vi "AI FSM.vi"(8 "Error In":errorcluster, 11 "Robot Mode":T1(ring)) -> (0 "Error Out":errorcluster, 1 "Heading_Cmd":dbl, 2 "VTan_Cmd":dbl, 3 "VAng_Cmd":dbl)   [LabVIEW 2012]
uses:
  Utilities/Robot Parameters/Robot Parameters.vi
panel:
  out "Bearing":dbl
  out "Target Distance":dbl
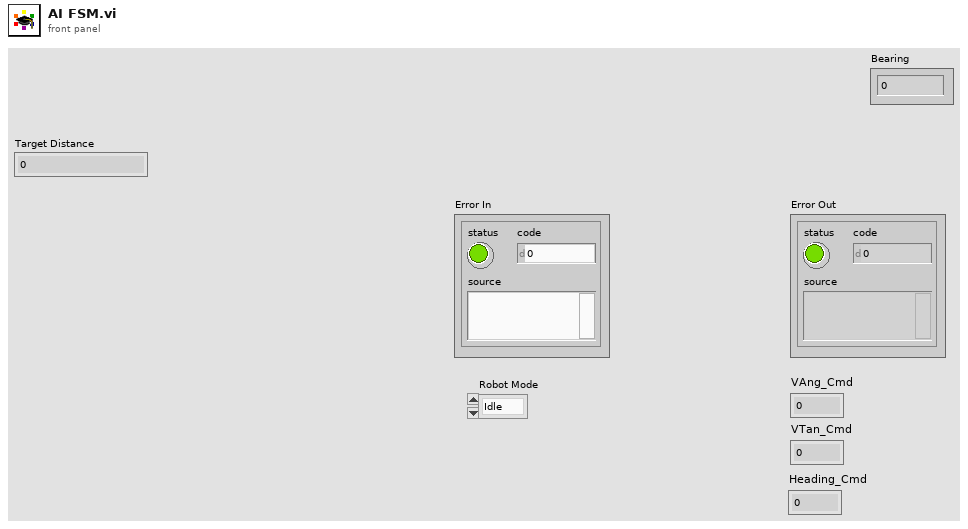
[diagram p1: front panel]
types:
  T1 = enum16{"Idle", "Wiimote", "Joypad", "IGVC", "Avoide Objects", "Avoide Lines", "Path Planning", "Heading", "Waypoint"}
  T2 = enum16{"Starting Line", "Line Following", "Waypoint Navigation", "Fence Hopping", "Finish Line", "Emergency"}
  T3 = cluster{"Latitude":dbl, "Longitude":dbl, "Altitude":dbl, "Velocity, Correction & SET":cluster{"Velocity North":dbl, "Velocity East":dbl, "Velocity Up":dbl, "Ellipsoidal Height":dbl, "GDOP":sgl, "PDOP":sgl, "HDOP":sgl, "VDOP":sgl, "TDOP":sgl, "Horizontal Figure of Merit":u8, "Time Figure of Merit":u8, "Max dGPS Age":sgl, "Extended Navigation Mode":u8, "Antenna Height Adjustment ":dbl, "SET North":i32, "SET East":i32, "SET Up":i32}, "Time":cluster{"GPS Week":u16, "GPS Time of Week":sgl}, "Satellites Used":i32[]}
  T4 = cluster{"Position":cluster{"Roll":dbl, "Pitch":dbl, "Yaw":dbl}, "Orientation Matrix":dbl[][], "Magnetic Field":cluster{"Z-Axis Magnetic Field":dbl, "Y-Axis Magnetic Field":dbl, "X-Axis Magnetic Field":dbl}, "Acceleration":cluster{"Z-Axis Acceleration":dbl, "Y-Axis Acceleration":dbl, "X-Axis Acceleration":dbl}, "Angular Rate":cluster{"X-Axis Angular Rate":dbl, "Y-Axis Angular Rate":dbl, "Z-Axis Angular Rate":dbl}, "Quaternion":dbl[]}
  T5 = cluster{"Latitude":dbl, "Longitude":dbl, "Altitude":dbl, "Velocity, Correction & SET":cluster{"Velocity North":dbl, "Velocity East":dbl, "Velocity Up":dbl, "Ellipsoidal Height":dbl, "GDOP":sgl, "PDOP":sgl, "HDOP":sgl, "VDOP":sgl, "TDOP":sgl, "Horizontal Figure of Merit":u8, "Time Figure of Merit":u8, "Max dGPS Age":sgl, "Extended Navigation Mode":u8, "Antenna Height Adjustment ":dbl, "SET North":i32, "SET East":i32, "SET Up":i32}, "Time":cluster{"GPS Week":u16, "GPS Time of Week":sgl}, "Satellites Used":i32[]}[]
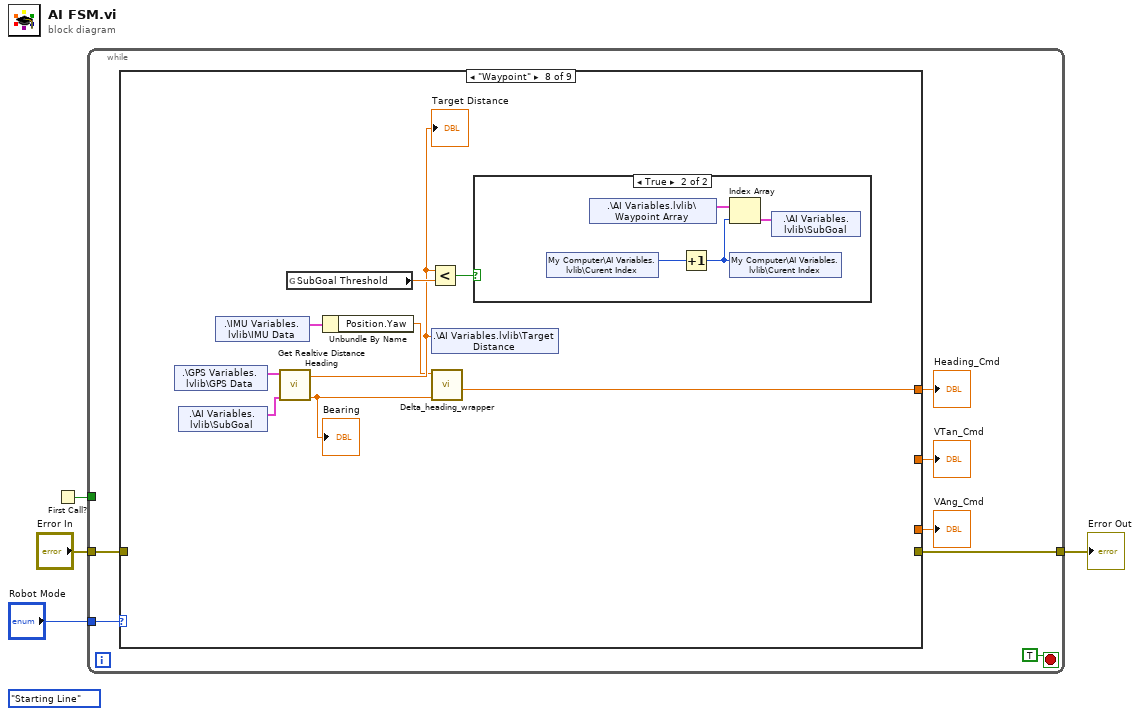
[diagram p0: block diagram]
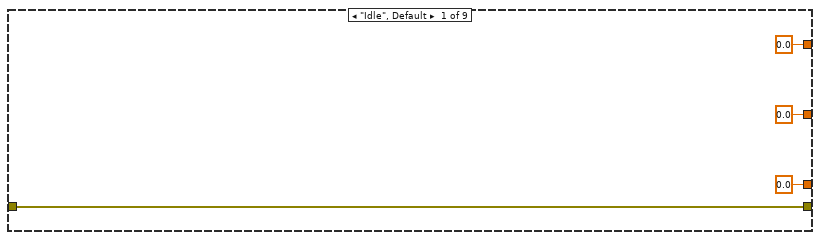
[diagram p2: hidden frame]
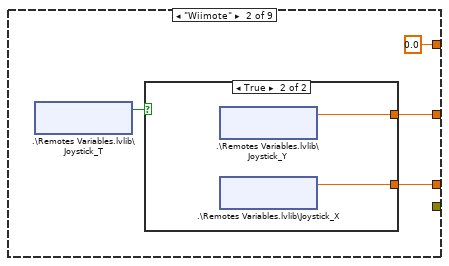
[diagram p3: hidden frame]
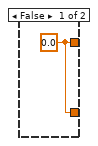
[diagram p4: hidden frame]
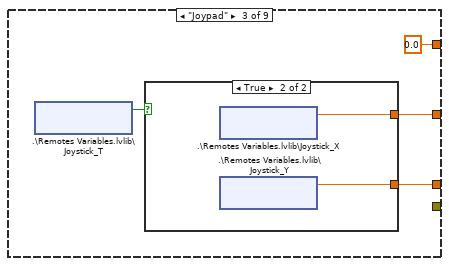
[diagram p5: hidden frame]
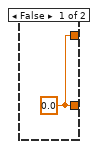
[diagram p6: hidden frame]
diagram:
  (unwired) T2."Starting Line" ("Enum")
  n1 = First Call?() -> (First Call?: T/F=w4:bool)
  n2 = while {
    tunnel: w4 -> [_]
    tunnel: "Error In" -> [w9]
    tunnel: [w8] -> w2
    tunnel: "Robot Mode" -> [w10]
    stop <- TRUE stop-if-true
    n3 = case shown="\"Waypoint\"" w10 {
      tunnel: [0.0 0.0 ("Numeric") 0.0 ("Numeric") _ _ _ _ w32 _] -> w5
      tunnel: [0.0 ("Double") w18 w23 _ _ _ _ _ _] -> w7
      tunnel: [0.0 w17 w25 _ _ _ _ _ _] -> w6
      tunnel: w9 -> [w13 _ _ _ _ _ _ _ _]
      tunnel: [w13 _ _ _ _ _ _ _ _] -> w8
      frame "Idle", Default {
      }
      frame "Wiimote" {
        n4 = shared-variable ".\\Remotes Variables.lvlib\\Joystick_T"() -> (w19:bool)  [unwired: 1 in, 2 out]
        n5 = case shown="True" w19 {
          tunnel: [w20 w22] -> w18
          tunnel: [w20 w21] -> w17
          frame False {
            w20 = 0.0
          }
          frame True {
            n6 = shared-variable ".\\Remotes Variables.lvlib\\Joystick_Y"() -> (w22:dbl)  [unwired: 1 in, 2 out]
            n7 = shared-variable ".\\Remotes Variables.lvlib\\Joystick_X"() -> (w21:dbl)  [unwired: 1 in, 2 out]
          }
        }
      }
      frame "Joypad" {
        n8 = shared-variable ".\\Remotes Variables.lvlib\\Joystick_T"() -> (w26:bool)  [unwired: 1 in, 2 out]
        n9 = case shown="True" w26 {
          tunnel: [w27 w29] -> w25
          tunnel: [w27 w28] -> w23
          frame False {
            w27 = 0.0
          }
          frame True {
            n10 = shared-variable ".\\Remotes Variables.lvlib\\Joystick_X"() -> (w28:dbl)  [unwired: 1 in, 2 out]
            n11 = shared-variable ".\\Remotes Variables.lvlib\\Joystick_Y"() -> (w29:dbl)  [unwired: 1 in, 2 out]
          }
        }
      }
      frame "IGVC" {
      }
      frame "Avoide Objects" {
      }
      frame "Avoide Lines" {
      }
      frame "Heading" {
      }
      frame "Waypoint" {
        n12 = shared-variable ".\\GPS Variables.lvlib\\GPS Data"() -> (w36:T3)  [unwired: 1 in, 1 out]
        n13 = shared-variable ".\\AI Variables.lvlib\\SubGoal"() -> (w35:T3)  [unwired: 1 in, 1 out]
        n14 = shared-variable ".\\IMU Variables.lvlib\\IMU Data"() -> (w37:T4)  [unwired: 1 in, 1 out]
        n15 = call "Get Realtive Distance Heading.vi"("Goal Position"=w35, "Current Position"=w36) -> ("Bearing"=w30:dbl, "distance (m)"=w34:dbl)  [unwired: 8 in]
        "Target Distance" <- w34
        "Bearing" <- w30
        n16 = global read "Robot Parameters.vi" "SubGoal Threshold"() -> (w38:dbl)
        n17 = Unbundle By Name(w37) -> ("Position.Yaw"=w31:dbl)
        n18 = Less?(x=w34, y=w38) -> (x < y?=w33:bool)
        n19 = shared-variable ".\\AI Variables.lvlib\\Target Distance"(w34) -> ()  [unwired: 1 in, 1 out]
        n20 = call "Delta_heading_wrapper.vi"("Goal Heading"=w30, "Robot Heading"=w31) -> ("Heading Adjustment"=w32:dbl)  [unwired: 9 in]
        n21 = case shown="True" w33 {
          frame False {
          }
          frame True {
            n22 = shared-variable "My Computer\\AI Variables.lvlib\\Curent Index"() -> (w42:i32)  [unwired: 1 in, 1 out]
            n23 = shared-variable ".\\AI Variables.lvlib\\Waypoint Array"() -> (w40:T5)  [unwired: 1 in, 1 out]
            n24 = Increment(x=w42) -> (x+1=w41:i32)
            n25 = Index Array(array=w40, index=w41) -> (element=w39:T3)
            n26 = shared-variable "My Computer\\AI Variables.lvlib\\Curent Index"(w41) -> ()  [unwired: 1 in, 1 out]
            n27 = shared-variable ".\\AI Variables.lvlib\\SubGoal"(w39) -> ()  [unwired: 1 in, 1 out]
          }
        }
      }
      frame "Path Planning" {
      }
    }
    "VAng_Cmd" <- w6
    "VTan_Cmd" <- w7
    "Heading_Cmd" <- w5
  }
  "Error Out" <- w2
